vi "TTA_MATLAB_RX_OutputPowerTest_DetailedResults.vi"(8 "error in":errorcluster, 9 "RxOutput\nPower Results":T1(array[cluster]), 10 "TestGroup":string, 11 "SubTest":string) -> (0 "error out":errorcluster, 3 "SubTestSuccess":dbl[](array[numeric]))   [LabVIEW 2016]
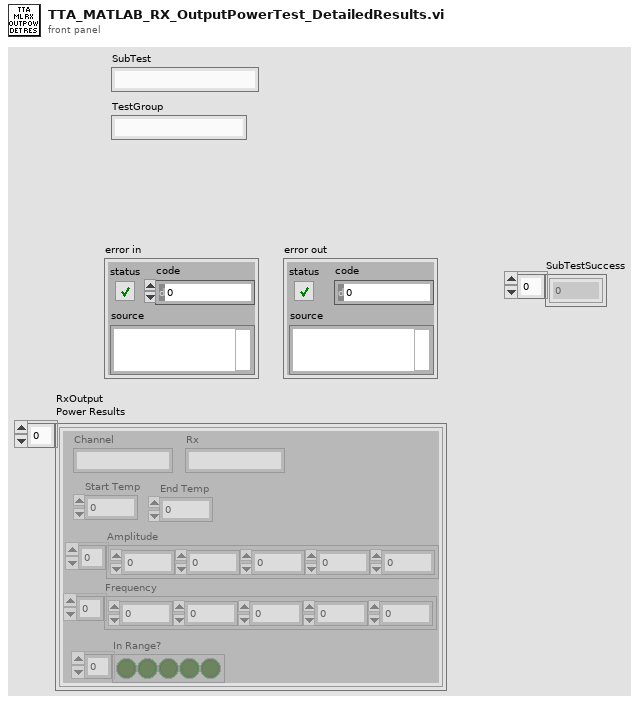
[diagram p1: front panel]
types:
  T1 = cluster{"Channel":string, "Rx":string, "Start Temp":dbl, "End Temp":dbl, "Amplitude":dbl[], "Frequency":dbl[], "In Range?":bool[]}[]
  T2 = cluster{"Channel":string, "Rx":string, "Start Temp":dbl, "End Temp":dbl, "Amplitude":dbl[], "Frequency":dbl[], "In Range?":bool[]}
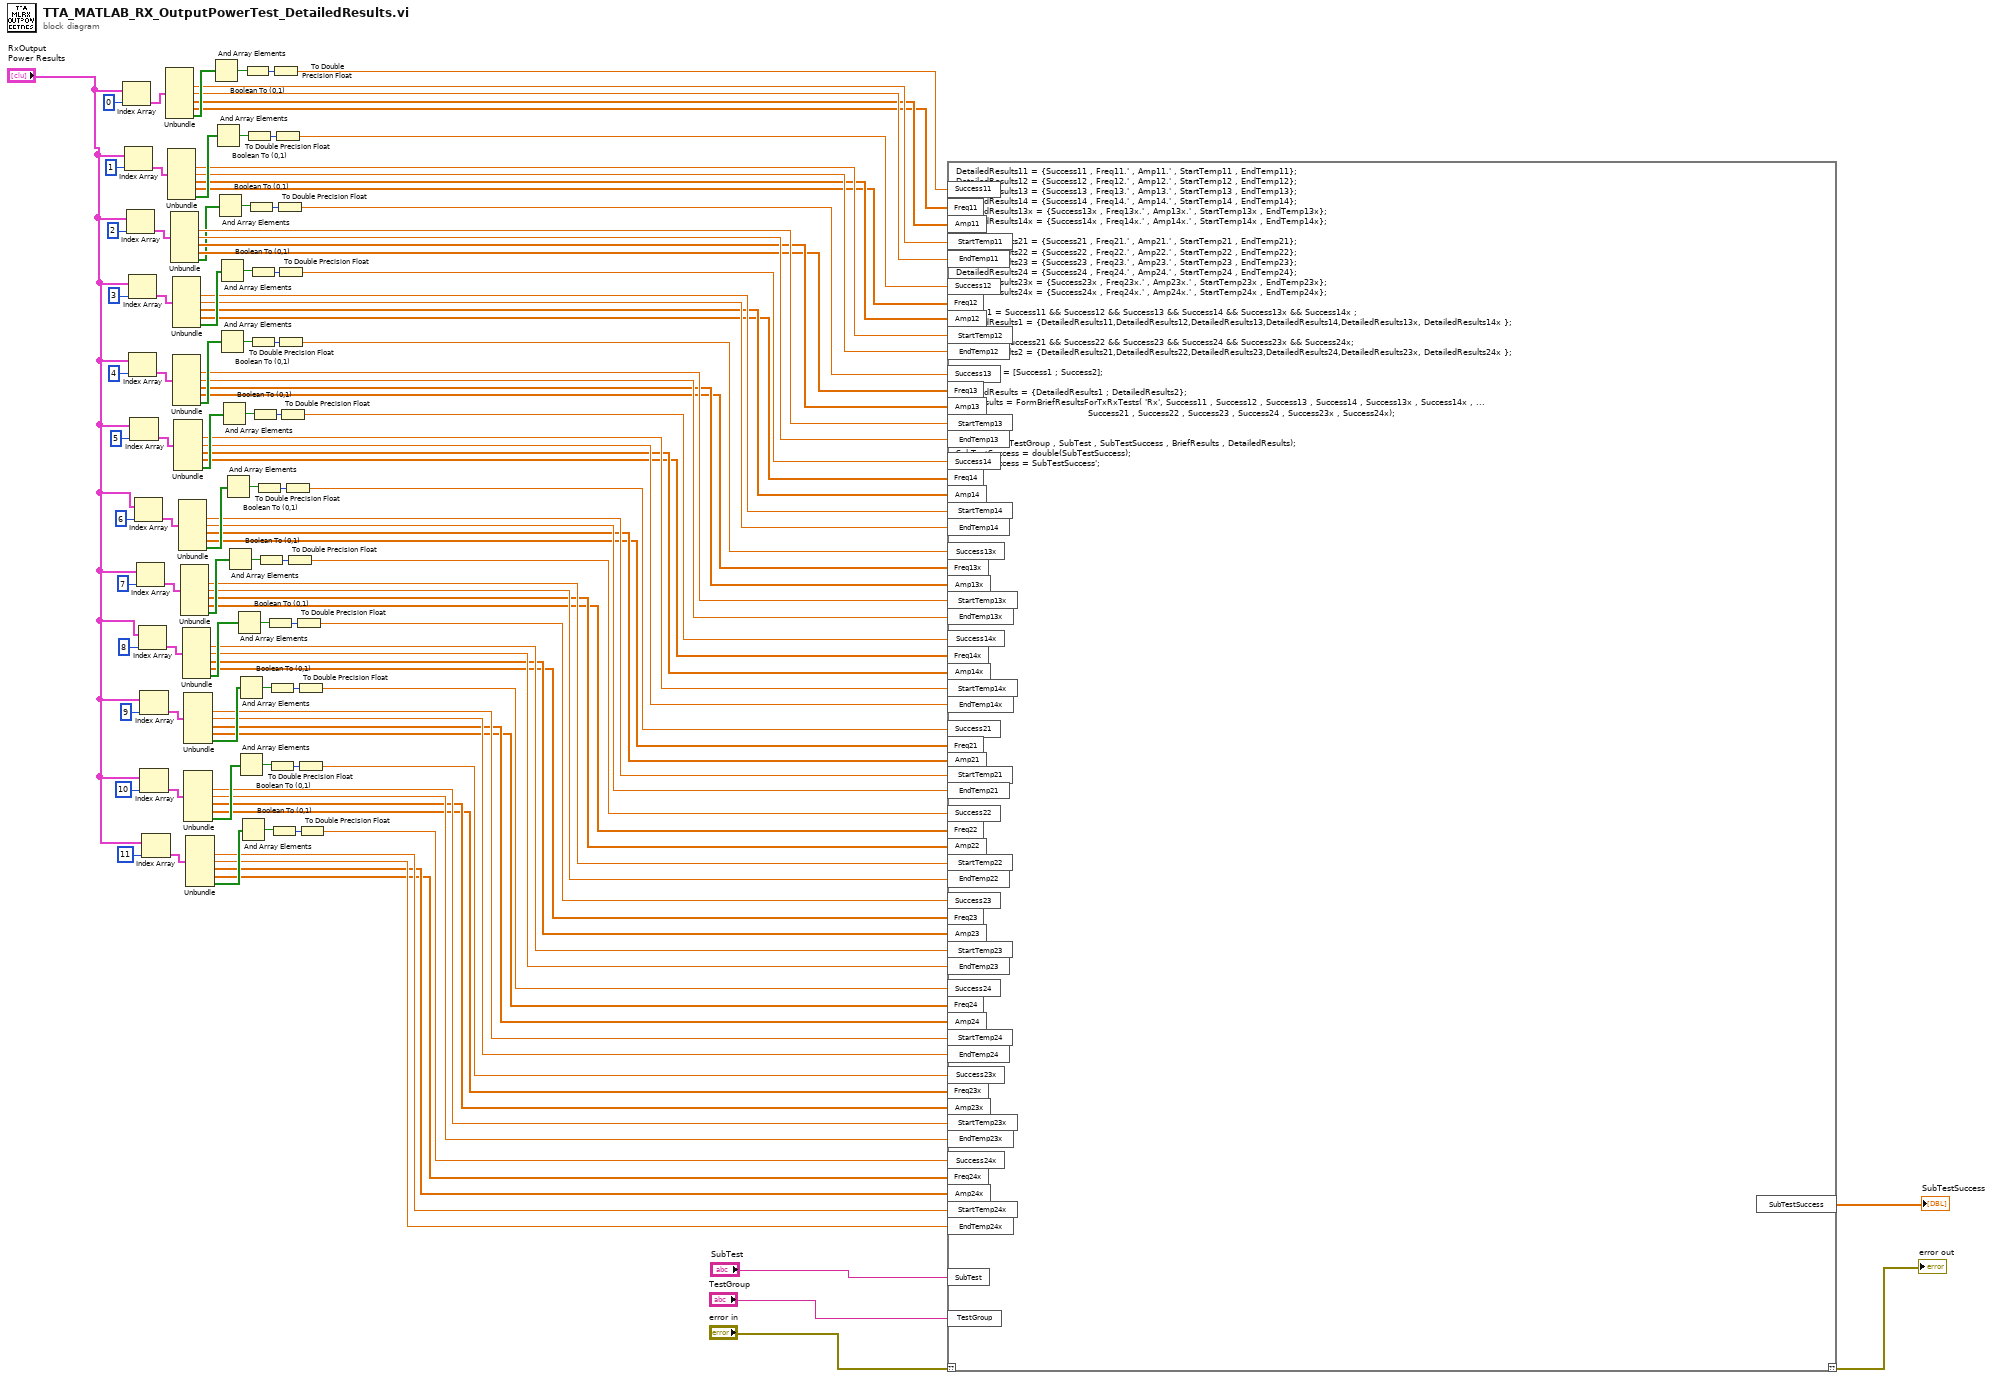
[diagram p0: block diagram]
diagram:
  (unwired) 5 ("index")
  (unwired) 3 ("index")
  (unwired) 2 ("index")
  (unwired) 1 ("index")
  (unwired) 0 ("index")
  (unwired) 5 ("index")
  (unwired) 4 ("index")
  (unwired) 3 ("index")
  (unwired) 2 ("index")
  (unwired) 1 ("index")
  (unwired) 0 ("index")
  (unwired) 5 ("index")
  (unwired) 4 ("index")
  (unwired) 3 ("index")
  (unwired) 2 ("index")
  (unwired) 1 ("index")
  (unwired) 0 ("index")
  (unwired) 5 ("index")
  (unwired) 4 ("index")
  (unwired) 3 ("index")
  (unwired) 2 ("index")
  (unwired) 1 ("index")
  (unwired) 0 ("index")
  (unwired) 4 ("index")
  n1 = Index Array(array="RxOutput\nPower Results", index=0) -> (element=w62:T2)
  n2 = Index Array(array="RxOutput\nPower Results", index=1) -> (element=w66:T2)
  n3 = Index Array(array="RxOutput\nPower Results", index=2) -> (element=w65:T2)
  n4 = Index Array(array="RxOutput\nPower Results", index=3) -> (element=w64:T2)
  n5 = Index Array(array="RxOutput\nPower Results", index=4) -> (element=w77:T2)
  n6 = Index Array(array="RxOutput\nPower Results", index=5) -> (element=w63:T2)
  n7 = Index Array(array="RxOutput\nPower Results", index=6) -> (element=w79:T2)
  n8 = Index Array(array="RxOutput\nPower Results", index=7) -> (element=w78:T2)
  n9 = Index Array(array="RxOutput\nPower Results", index=8) -> (element=w74:T2)
  n10 = Index Array(array="RxOutput\nPower Results", index=9) -> (element=w72:T2)
  n11 = Index Array(array="RxOutput\nPower Results", index=10) -> (element=w71:T2)
  n12 = Index Array(array="RxOutput\nPower Results", index=11) -> (element=w70:T2)
  n13 = Unbundle(w62) -> ("Start Temp"=w59:dbl, "End Temp"=w58:dbl, "Amplitude"=w57:dbl[], "Frequency"=w56:dbl[], "In Range?"=w60:bool[])  [unwired: 2 out]
  n14 = Unbundle(w66) -> ("Start Temp"=w54:dbl, "End Temp"=w53:dbl, "Amplitude"=w52:dbl[], "Frequency"=w51:dbl[], "In Range?"=w55:bool[])  [unwired: 2 out]
  n15 = Unbundle(w65) -> ("Start Temp"=w50:dbl, "End Temp"=w49:dbl, "Amplitude"=w48:dbl[], "Frequency"=w47:dbl[], "In Range?"=w46:bool[])  [unwired: 2 out]
  n16 = Unbundle(w64) -> ("Start Temp"=w44:dbl, "End Temp"=w43:dbl, "Amplitude"=w42:dbl[], "Frequency"=w41:dbl[], "In Range?"=w45:bool[])  [unwired: 2 out]
  n17 = Unbundle(w77) -> ("Start Temp"=w39:dbl, "End Temp"=w38:dbl, "Amplitude"=w37:dbl[], "Frequency"=w36:dbl[], "In Range?"=w40:bool[])  [unwired: 2 out]
  n18 = Unbundle(w63) -> ("Start Temp"=w34:dbl, "End Temp"=w33:dbl, "Amplitude"=w32:dbl[], "Frequency"=w31:dbl[], "In Range?"=w35:bool[])  [unwired: 2 out]
  n19 = Unbundle(w79) -> ("Start Temp"=w29:dbl, "End Temp"=w28:dbl, "Amplitude"=w27:dbl[], "Frequency"=w26:dbl[], "In Range?"=w30:bool[])  [unwired: 2 out]
  n20 = Unbundle(w78) -> ("Start Temp"=w24:dbl, "End Temp"=w23:dbl, "Amplitude"=w22:dbl[], "Frequency"=w21:dbl[], "In Range?"=w25:bool[])  [unwired: 2 out]
  n21 = Unbundle(w74) -> ("Start Temp"=w19:dbl, "End Temp"=w18:dbl, "Amplitude"=w17:dbl[], "Frequency"=w16:dbl[], "In Range?"=w20:bool[])  [unwired: 2 out]
  n22 = Unbundle(w72) -> ("Start Temp"=w14:dbl, "End Temp"=w13:dbl, "Amplitude"=w12:dbl[], "Frequency"=w11:dbl[], "In Range?"=w15:bool[])  [unwired: 2 out]
  n23 = Unbundle(w71) -> ("Start Temp"=w9:dbl, "End Temp"=w8:dbl, "Amplitude"=w7:dbl[], "Frequency"=w6:dbl[], "In Range?"=w10:bool[])  [unwired: 2 out]
  n24 = Unbundle(w70) -> ("Start Temp"=w4:dbl, "End Temp"=w3:dbl, "Amplitude"=w2:dbl[], "Frequency"=w1:dbl[], "In Range?"=w5:bool[])  [unwired: 2 out]
  n25 = And Array Elements(Boolean array=w60) -> (logical AND=w120:bool)
  n26 = And Array Elements(Boolean array=w55) -> (logical AND=w116:bool)
  n27 = And Array Elements(Boolean array=w46) -> (logical AND=w109:bool)
  n28 = And Array Elements(Boolean array=w45) -> (logical AND=w112:bool)
  n29 = And Array Elements(Boolean array=w40) -> (logical AND=w107:bool)
  n30 = And Array Elements(Boolean array=w35) -> (logical AND=w104:bool)
  n31 = And Array Elements(Boolean array=w30) -> (logical AND=w81:bool)
  n32 = And Array Elements(Boolean array=w25) -> (logical AND=w84:bool)
  n33 = And Array Elements(Boolean array=w20) -> (logical AND=w90:bool)
  n34 = And Array Elements(Boolean array=w15) -> (logical AND=w87:bool)
  n35 = And Array Elements(Boolean array=w10) -> (logical AND=w93:bool)
  n36 = And Array Elements(Boolean array=w5) -> (logical AND=w96:bool)
  n37 = Boolean To (0,1)(Boolean=w120) -> (0, 1=w119:i16)
  n38 = Boolean To (0,1)(Boolean=w116) -> (0, 1=w117:i16)
  n39 = Boolean To (0,1)(Boolean=w109) -> (0, 1=w110:i16)
  n40 = Boolean To (0,1)(Boolean=w112) -> (0, 1=w111:i16)
  n41 = Boolean To (0,1)(Boolean=w107) -> (0, 1=w106:i16)
  n42 = Boolean To (0,1)(Boolean=w104) -> (0, 1=w105:i16)
  n43 = Boolean To (0,1)(Boolean=w81) -> (0, 1=w82:i16)
  n44 = Boolean To (0,1)(Boolean=w84) -> (0, 1=w83:i16)
  n45 = Boolean To (0,1)(Boolean=w90) -> (0, 1=w89:i16)
  n46 = Boolean To (0,1)(Boolean=w87) -> (0, 1=w88:i16)
  n47 = Boolean To (0,1)(Boolean=w93) -> (0, 1=w94:i16)
  n48 = Boolean To (0,1)(Boolean=w96) -> (0, 1=w95:i16)
  n49 = To Double Precision Float(number=w119) -> (double precision float=w118:dbl)
  n50 = To Double Precision Float(number=w117) -> (double precision float=w114:dbl)
  n51 = To Double Precision Float(number=w110) -> (double precision float=w102:dbl)
  n52 = To Double Precision Float(number=w111) -> (double precision float=w101:dbl)
  n53 = To Double Precision Float(number=w106) -> (double precision float=w100:dbl)
  n54 = To Double Precision Float(number=w105) -> (double precision float=w99:dbl)
  n55 = To Double Precision Float(number=w82) -> (double precision float=w76:dbl)
  n56 = To Double Precision Float(number=w83) -> (double precision float=w75:dbl)
  n57 = To Double Precision Float(number=w89) -> (double precision float=w73:dbl)
  n58 = To Double Precision Float(number=w88) -> (double precision float=w69:dbl)
  n59 = To Double Precision Float(number=w94) -> (double precision float=w68:dbl)
  n60 = To Double Precision Float(number=w95) -> (double precision float=w67:dbl)
  n61 = script code="DetailedResults11 = {Success11 , Freq11.' , Amp11.' , StartTemp11 , EndTemp11};\nDetailedResults12 = {Success12 , Freq12.' , Amp12.' , StartTemp12 , EndTemp12};\nDetailedResults13 = {Success13 , Freq13.' , Amp13.' , StartTemp13 , EndTemp13};\nDetailedResults14 = {Success14 , Freq14.' , Amp14.' , StartTemp14 , EndTemp14};\nDetailedResults13x = {Success13x , Freq13x.' , Amp13x.' , StartTemp13x , EndTemp13x};\nDetailedResults14x = {Success14x , Freq14x.' , Amp14x.' , StartTemp14x , EndTemp14x};\n\nDetailedResults21 = {Success21 , Freq21.' , Amp21.' , StartTemp21 , EndTemp21};\nDetailedResults22 = {Success22 , Freq22.' , Amp22.' , StartTemp22 , EndTemp22};\nDetailedResults23 = {Success23 , Freq23.' , Amp23.' , StartTemp23 , EndTemp23};\nDetailedResults24 = {Success24 , Freq24.' , Amp24.' , StartTemp24 , EndTemp24};\nDetailedResults23x = {Success23x , Freq23x.' , Amp23x.' , StartTemp23x , EndTemp23x};\nDetailedResults24x = {Success24x , Freq24x.' , Amp24x.' , StartTemp24x , EndTemp24x};\n\nSuccess1 = Success11 && Success12 && Success13 && Success14 && Success13x && Success14x ;\nDetailedResults1 = {DetailedResults11,DetailedResults12,DetailedResults13,DetailedResults14,DetailedResults13x, DetailedResults14x };\n\nSuccess2 = Success21 && Success22 && Success23 && Success24 && Success23x && Success24x;\nDetailedResults2 = {DetailedResults21,DetailedResults22,DetailedResults23,DetailedResults24,DetailedResults23x, DetailedResults24x };\n\nSuccessList = [Success1 ; Success2];\n\nDetailedResults = {DetailedResults1 ; DetailedResults2};\nBriefResults = FormBriefResultsForTxRxTests( 'Rx', Success11 , Success12 , Success13 , Success14 , Success13x , Success14x , ...\n                                            Success21 , Success22 , Success23 , Success24 , Success23x , Success24x);\n\n\nUpdateState(TestGroup , SubTest , SubTestSuccess , BriefResults , DetailedResults);\nSubTestSuccess = double(SubTestSuccess);\nSubTestSuccess = SubTestSuccess';"("??"="error in", "SubTest"="SubTest", "TestGroup"="TestGroup", "Success11"=w118, "Freq11"=w56, "Amp11"=w57, "StartTemp11"=w59, "EndTemp11"=w58, "Success12"=w114, "Freq12"=w51, "Amp12"=w52, "StartTemp12"=w54, "EndTemp12"=w53, "Success13"=w102, "Freq13"=w47, "Amp13"=w48, "StartTemp13"=w50, "EndTemp13"=w49, "Success14"=w101, "Freq14"=w41, "Amp14"=w42, "StartTemp14"=w44, "EndTemp14"=w43, "Success13x"=w100, "Freq13x"=w36, "Amp13x"=w37, "StartTemp13x"=w39, "EndTemp13x"=w38, "Success14x"=w99, "Freq14x"=w31, "Amp14x"=w32, "StartTemp14x"=w34, "EndTemp14x"=w33, "Success21"=w76, "Freq21"=w26, "Amp21"=w27, "StartTemp21"=w29, "EndTemp21"=w28, "Success22"=w75, "Freq22"=w21, "Amp22"=w22, "StartTemp22"=w24, "EndTemp22"=w23, "Success23"=w73, "Freq23"=w16, "Amp23"=w17, "StartTemp23"=w19, "EndTemp23"=w18, "Success24"=w69, "Freq24"=w11, "Amp24"=w12, "StartTemp24"=w14, "EndTemp24"=w13, "Success23x"=w68, "Freq23x"=w6, "Amp23x"=w7, "StartTemp23x"=w9, "EndTemp23x"=w8, "Success24x"=w67, "Freq24x"=w1, "Amp24x"=w2, "StartTemp24x"=w4, "EndTemp24x"=w3) -> ("??"=→"error out":errorcluster, "SubTestSuccess"=→"SubTestSuccess":dbl[])
